vi "IndoorData_Init.vi"(0 "reference in":refnum<class "IndoorData.lvclass"> caption="This control should only be used when\na sub class is inheriting this class", 5 "error in (no error)":errorcluster) -> (14 "reference out":refnum<class "IndoorData.lvclass"> caption="This indicator should only be used when\na sub class is inheriting this class", 19 "error out":errorcluster)   [LabVIEW 2019, in "IndoorData.lvclass"]
uses:
  IndoorData.lvclass
  DebugData.ctl
  ActualValues.ctl
  BufferedReadings.ctl
  <vilib>/MakerHub/Toolbox/LMH-Toolbox.lvlib
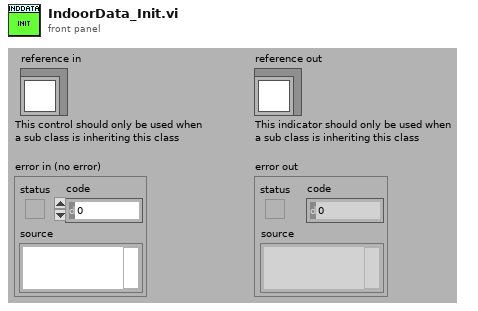
[diagram p1: front panel]
types:
  T1 = typedef "IndoorData.lvclass/BufferedReadings.ctl" = cluster{"Time":dbl[], "Temp":dbl[], "RH":dbl[]}
  T2 = typedef "IndoorData.lvclass/ActualValues.ctl" = cluster{"Time":dbl, "Temp":dbl, "RH":dbl}
  T3 = typedef "IndoorData.lvclass/DebugData.ctl" = cluster{"Rev":string, "Location":string, "LoopIdx":i32, "PiCoreTemp":dbl, "Error":errorcluster}
  T4 = typedef "IndoorData.lvclass/ObjectAttributes.ctl" = cluster{"DebugData":T3, "Actual":T2, "BufferedReadings":T1, "AVGReadings":T1, "LogFolder":path, "FirstLog?":bool, "MinMaxFile":path}
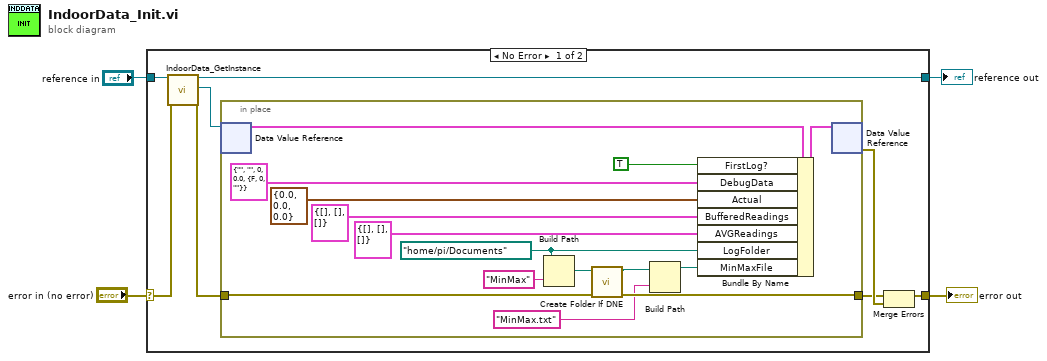
[diagram p0: block diagram]
diagram:
  n1 = case shown="No Error" "error in (no error)" {
    selector: "error in (no error)" -> [w10 w29]
    tunnel: [w11 w29] -> w3
    tunnel: "reference in" -> [w9 w28]
    tunnel: [w8 w28] -> w1
    frame No Error {
      n2 = call "IndoorData_GetInstance.vi"("reference in"=w9, "error in (no error)"=w10) -> ("reference out"=w8:refnum<class "IndoorData.lvclass">, "DVRRefOut"=w7:refnum<data-value>, "error out"=w5:errorcluster)  [unwired: 13 in, 2 out]
      n3 = in-place {
        in-place-border: w5 -> [w17]
        in-place-border: [w16] -> w6
        w20 = path "/home/pi/Documents"
        n4 = in-place-dvr #1(w7) -> (w26:T4)  [unwired: 1 out]
        n5 = Build Path(base path=w20, name or relative path="MinMax") -> (appended path=w18:path)
        n6 = call <vilib>:"Create Folder If DNE.vi"("Error In"=w17, "Folder Path"=w18) -> ("Error Out"=w16:errorcluster, "Dup Path"=w15:path)  [unwired: 8 in]
        n7 = Build Path(base path=w15, name or relative path="MinMax.txt") -> (appended path=w14:path)
        n8 = Bundle By Name(cluster=w26, "FirstLog?"=TRUE ("Reboot?"), "DebugData"=T3 {"Rev"="", "Location"="", "LoopIdx"=0, "PiCoreTemp"=0.0, "Error"={"status"=FALSE, "code"=0, "source"=""}}, "Actual"=T2 {"Time"=0.0, "Temp"=0.0, "RH"=0.0}, "BufferedReadings"=T1 {"Time"=[], "Temp"=[], "RH"=[]}, "AVGReadings"=T1 {"Time"=[], "Temp"=[], "RH"=[]}, "LogFolder"=w20, "MinMaxFile"=w14) -> (w27:T4)
        n9 = in-place-dvr #1(w27) -> (w12:errorcluster)  [unwired: 1 out]
      }
      n10 = Merge Errors(w6, w12) -> (w11:errorcluster)
    }
    frame Error {
    }
  }
  "error out" <- w3
  "reference out" <- w1
